vi "函数类型1测试 - 副本.vi"() -> ()   [LabVIEW 2010]
uses:
  全局量/试验配置信息.vi
panel:
  out "bRece":bool
  out "bSend":bool
  out "D_IN_1":string[][](table) caption="表格"
  in  "加载文件名称":string
  out "配置文件路径":path
  out "配置文件目录":path
  in  "同步_1":i32
  in  "数组_反馈值":dbl[][](array[numeric])
  in  "第几个数据":i32
  in  "第几组数据":i32
  in  "数组_设定值":dbl[][](array[numeric])
  in  "数组_选择":bool[](array[boolean])
  out "light_32":bool
  out "light_31":bool
  out "light_30":bool
  out "light_29":bool
  out "light_28":bool
  out "light_27":bool
  out "light_26":bool
  out "light_25":bool
  out "light_24":bool
  out "light_23":bool
  out "light_22":bool
  out "light_21":bool
  out "light_20":bool
  out "light_19":bool
  out "light_18":bool
  out "light_17":bool
  out "Analog_back":string[][](table) caption="表格"
  in  "A_32":bool
  in  "A_31":bool
  in  "A_30":bool
  in  "A_29":bool
  in  "A_28":bool
  in  "A_27":bool
  in  "A_26":bool
  in  "A_25":bool
  in  "A_24":bool
  in  "A_23":bool
  in  "A_22":bool
  in  "A_21":bool
  in  "A_20":bool
  in  "A_19":bool
  in  "A_18":bool
  in  "A_17":bool
  out "合格？":bool[][](array[boolean])
  out "测试结论":string
  out "light_16":bool
  out "light_15":bool
  out "light_14":bool
  out "light_13":bool
  out "light_12":bool
  out "light_11":bool
  out "light_10":bool
  out "light_9":bool
  out "light_8":bool
  out "light_7":bool
  out "light_6":bool
  out "light_5":bool
  out "light_4":bool
  out "light_3":bool
  out "light_2":bool
  out "light_1":bool
  out "退出？":bool
  in  "btn_反选":bool
  in  "btn_全选":bool
  in  "A_16":bool
  in  "A_15":bool
  in  "A_14":bool
  in  "A_13":bool
  in  "A_12":bool
  in  "A_11":bool
  in  "A_10":bool
  in  "A_9":bool
  in  "A_8":bool
  in  "A_7":bool
  in  "A_6":bool
  in  "A_5":bool
  in  "A_4":bool
  in  "A_3":bool
  in  "A_2":bool
  in  "A_1":bool
  in  "btn_取消":bool
  in  "btn_开始测试":bool
  in  "Analog_IN":string[][](table) caption="表格"
  out "Analog_WC":string[][](table) caption="表格"
  # "模拟量选择及输入值（V）"
  # "模拟量反馈值（V）"
  # "模拟量误差值（%）"
  # "测试结论："
  # "从0开始"
  # "从1开始,第0列没有使用"
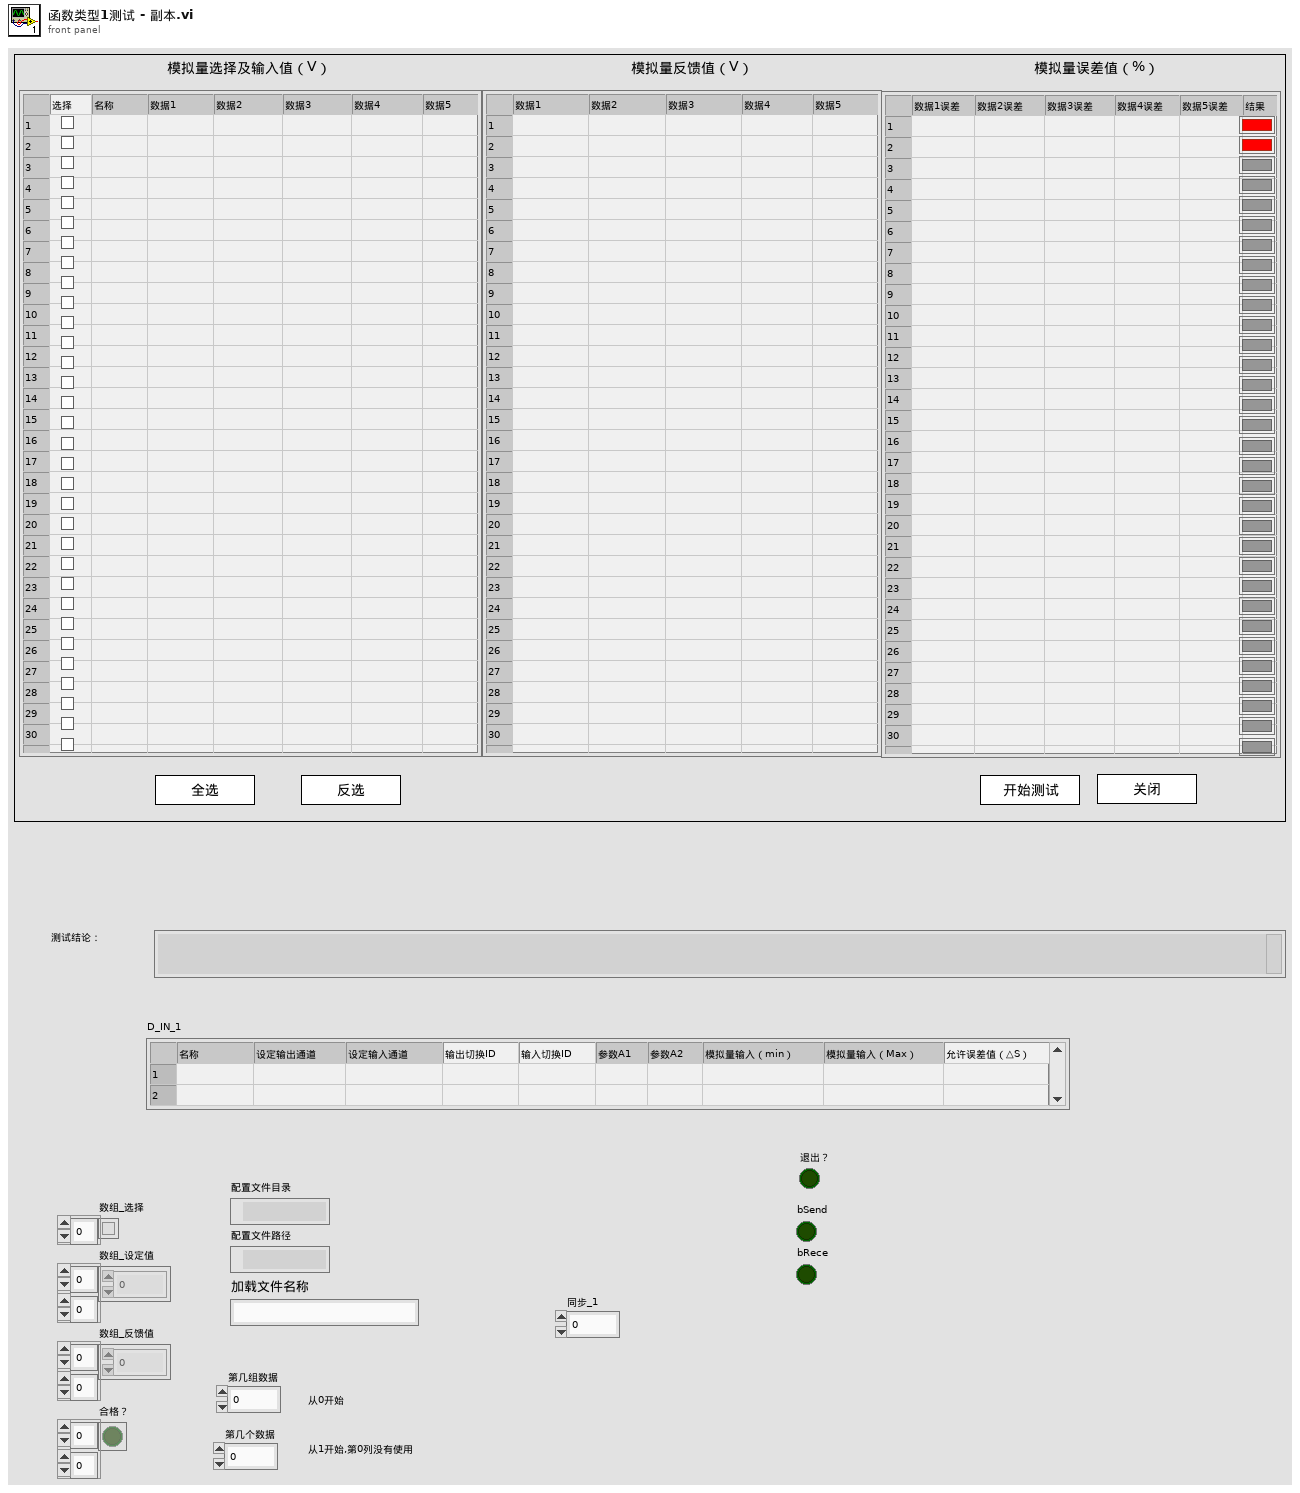
[diagram p1: front panel]
types:
  T1 = enum8{"Enabled", "Disabled", "Disabled and Grayed Out"}
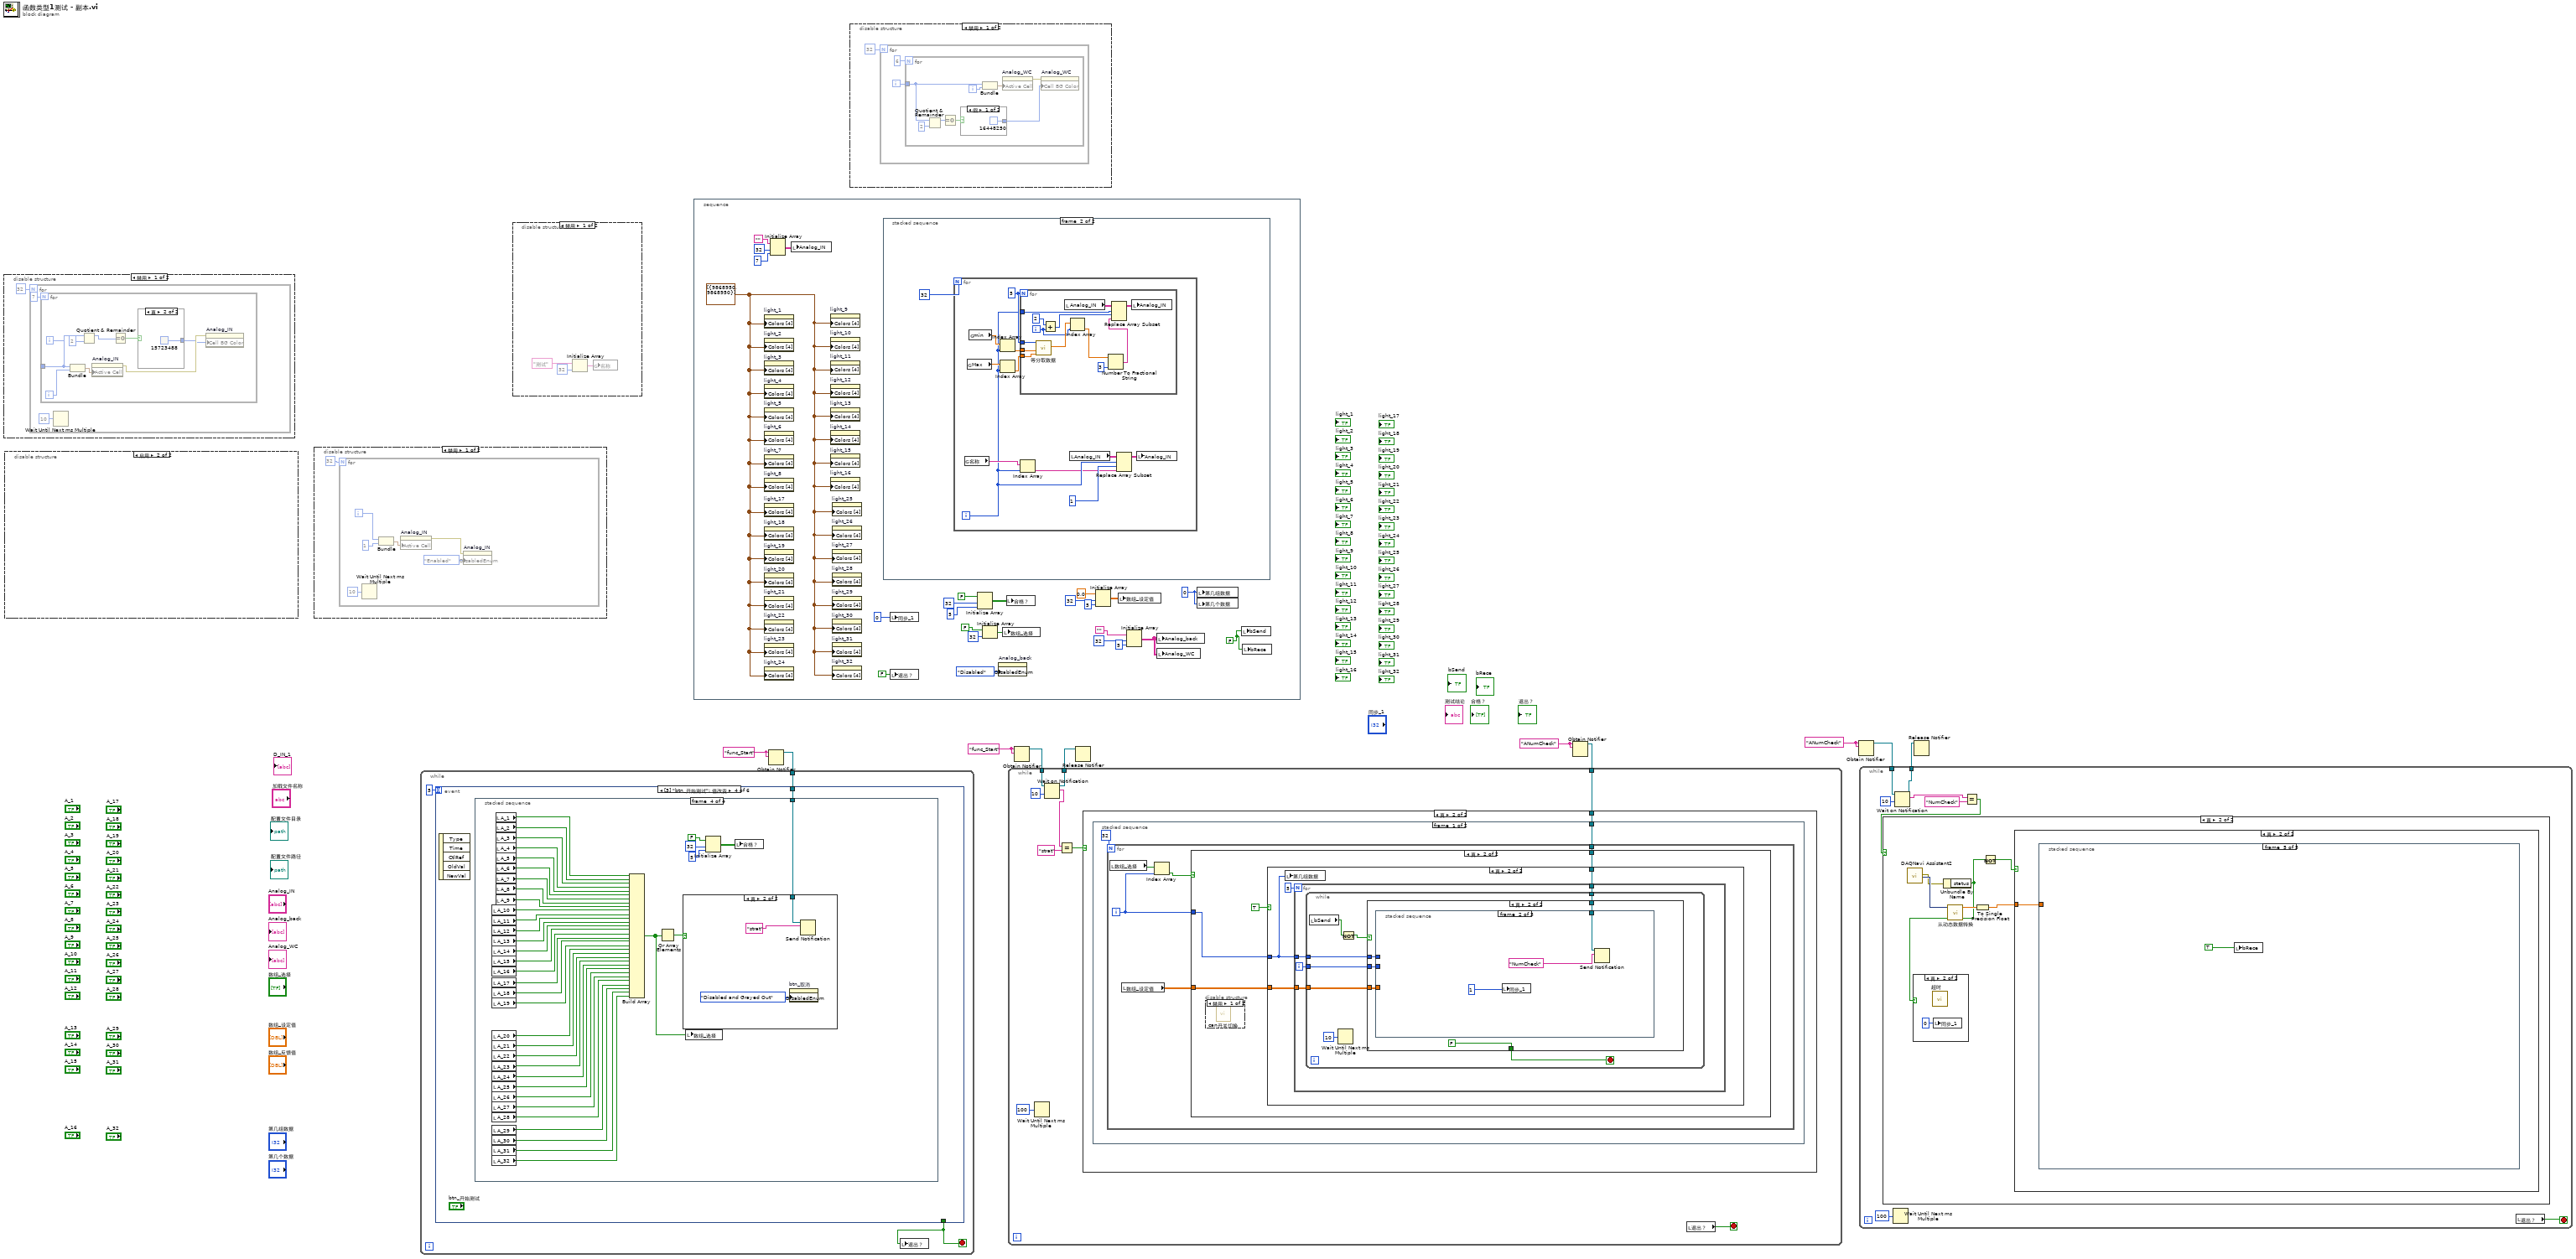
[diagram p0: block diagram]
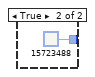
[diagram p2: hidden frame]
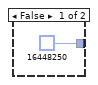
[diagram p5: hidden frame]
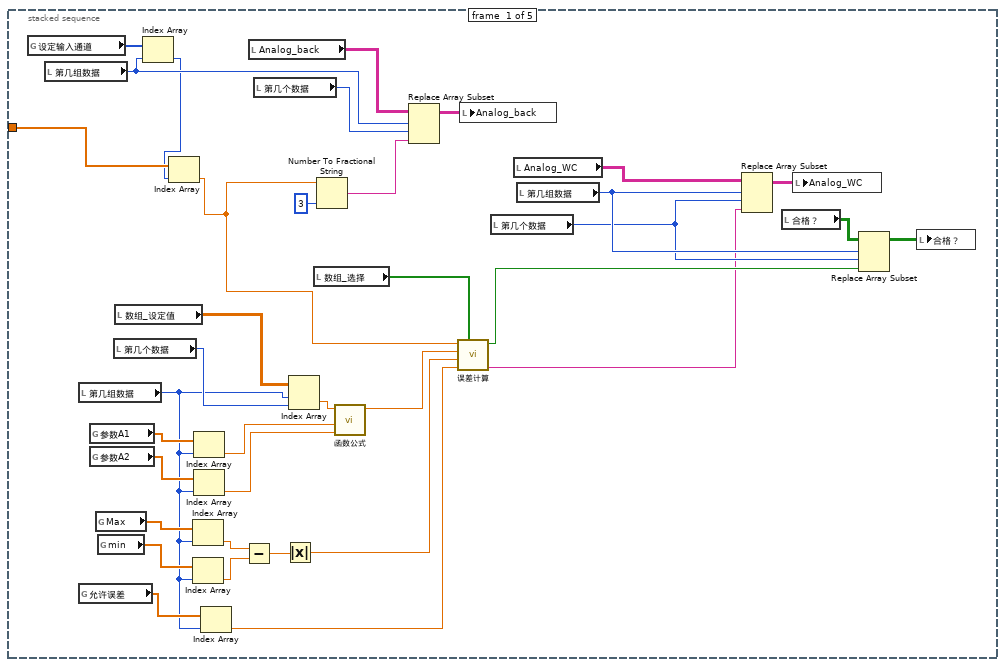
[diagram p10: hidden frame]
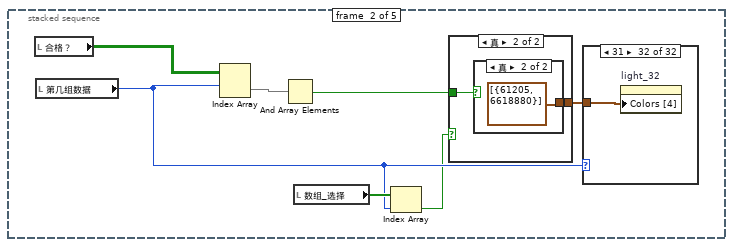
[diagram p11: hidden frame]
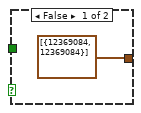
[diagram p12: hidden frame]
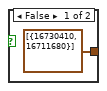
[diagram p13: hidden frame]
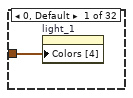
[diagram p14: hidden frame]
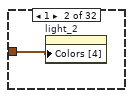
[diagram p15: hidden frame]
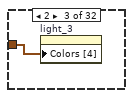
[diagram p16: hidden frame]
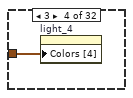
[diagram p17: hidden frame]
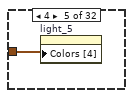
[diagram p18: hidden frame]
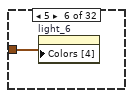
[diagram p19: hidden frame]
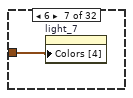
[diagram p20: hidden frame]
diagram:
  w2 = "ANumCheck" ("名称（未命名）")
  w4 = "func_Start" ("名称（未命名）")
  w8 = "ANumCheck" ("名称（未命名）")
  w10 = "func_Start" ("名称（未命名）")
  n1 = disable-structure shown="禁用" {
    frame Disabled {
      n2 = for {
        N: 32 -> [_]
        i -> [w13]
        n3 = for {
          N: 7 -> [_]
          tunnel: w13 -> [w21]
          i -> [w15]
          n4 = Bundle(w21, w15) -> (w18:cluster{i32, i32})  [unwired: 1 in]
          n5 = Quotient & Remainder(x=w21, y=2) -> (x-y*floor(x/y)=w19:i32)  [unwired: 1 out]
          n6 = property on="Analog_IN" class="Tbl (严格)"("Active Cell"=w18) -> (error out=w17:errorcluster)  [unwired: 2 in, 1 out]
          n7 = Equal To 0?(x=w19) -> (x = 0?=w22:bool)
          n8 = case shown="真" w22 {
            tunnel: [u32 16448250 u32 15723488] -> w16
            frame False {
            }
            frame True {
            }
          }
          n9 = property on="Analog_IN" class="Tbl (严格)"(error in=w17, "Cell BG Color"=w16) -> ()  [unwired: 1 in, 2 out]
        }
        n10 = Wait Until Next ms Multiple(millisecond multiple=u32 10 ("毫秒倍数")) -> ()  [unwired: 1 out]
      }
    }
    frame Enabled {
    }
  }
  n11 = disable-structure shown="启用" {
    frame Disabled {
      n12 = for {
        N: 32 -> [_]
        i -> [w26]
        n13 = for {
          N: 7 -> [_]
          tunnel: w26 -> [w29]
          i -> [w30]
          n14 = Bundle(w29, w30) -> (w33:cluster{i32, i32})  [unwired: 1 in]
          n15 = property on="Analog_IN" class="Tbl (严格)"("Active Cell"=w33) -> (error out=w31:errorcluster)  [unwired: 2 in, 1 out]
          n16 = property on="Analog_IN" class="Tbl (严格)"(error in=w31, "Justify"=enum16{"Left", "Center", "Right"}."Left" ("活动单元格:单元格对齐")) -> ()  [unwired: 1 in, 2 out]
        }
        n17 = Wait Until Next ms Multiple(millisecond multiple=u32 10 ("毫秒倍数")) -> ()  [unwired: 1 out]
      }
    }
    frame Enabled {
    }
  }
  n18 = disable-structure shown="禁用" {
    frame Disabled {
      n19 = for {
        N: 32 -> [_]
        i -> [w39]
        n20 = Wait Until Next ms Multiple(millisecond multiple=u32 10 ("毫秒倍数")) -> ()  [unwired: 1 out]
        n21 = Bundle(w39, 1) -> (w38:cluster{i32, i32})  [unwired: 1 in]
        n22 = property on="Analog_IN" class="Tbl (严格)"("Active Cell"=w38) -> (error out=w35:errorcluster)  [unwired: 2 in, 1 out]
        n23 = property on="Analog_IN" class="Tbl (严格)"(error in=w35, "DisabledEnum"=T1."Enabled" ("禁用")) -> ()  [unwired: 1 in, 2 out]
      }
    }
    frame Enabled {
    }
  }
  n24 = disable-structure shown="禁用" {
    frame Disabled {
      n25 = Initialize Array("测试", 32 ("维数大小")) -> (w42:string[])
      n26 = global write "试验配置信息.vi" "名称"(w42) -> ()
    }
    frame Enabled {
    }
  }
  n27 = stacked-sequence {
    frame #0 {
      w44 = FALSE
      w49 = 0 ("第几组数据")
      w64 = cluster{u32, u32}[] [{9868950, 9868950}]
      n28 = property on="light_1" class="Bool (严格)"("Colors [4]"=w64) -> ()  [unwired: 2 in, 2 out]
      n29 = property on="light_2" class="Bool (严格)"("Colors [4]"=w64) -> ()  [unwired: 2 in, 2 out]
      n30 = property on="light_3" class="Bool (严格)"("Colors [4]"=w64) -> ()  [unwired: 2 in, 2 out]
      n31 = property on="light_4" class="Bool (严格)"("Colors [4]"=w64) -> ()  [unwired: 2 in, 2 out]
      n32 = property on="light_5" class="Bool (严格)"("Colors [4]"=w64) -> ()  [unwired: 2 in, 2 out]
      n33 = property on="light_6" class="Bool (严格)"("Colors [4]"=w64) -> ()  [unwired: 2 in, 2 out]
      n34 = property on="light_7" class="Bool (严格)"("Colors [4]"=w64) -> ()  [unwired: 2 in, 2 out]
      n35 = property on="light_8" class="Bool (严格)"("Colors [4]"=w64) -> ()  [unwired: 2 in, 2 out]
      n36 = property on="light_17" class="Bool (严格)"("Colors [4]"=w64) -> ()  [unwired: 2 in, 2 out]
      n37 = property on="light_18" class="Bool (严格)"("Colors [4]"=w64) -> ()  [unwired: 2 in, 2 out]
      n38 = property on="light_19" class="Bool (严格)"("Colors [4]"=w64) -> ()  [unwired: 2 in, 2 out]
      n39 = property on="light_20" class="Bool (严格)"("Colors [4]"=w64) -> ()  [unwired: 2 in, 2 out]
      n40 = property on="light_21" class="Bool (严格)"("Colors [4]"=w64) -> ()  [unwired: 2 in, 2 out]
      n41 = property on="light_22" class="Bool (严格)"("Colors [4]"=w64) -> ()  [unwired: 2 in, 2 out]
      n42 = property on="light_23" class="Bool (严格)"("Colors [4]"=w64) -> ()  [unwired: 2 in, 2 out]
      n43 = property on="light_24" class="Bool (严格)"("Colors [4]"=w64) -> ()  [unwired: 2 in, 2 out]
      n44 = Initialize Array("", 32 ("维数大小"), 7 ("维数大小")) -> (w48:string[][])
      n45 = local write "Analog_IN"(w48) -> ()
      n46 = property on="light_9" class="Bool (严格)"("Colors [4]"=w64) -> ()  [unwired: 2 in, 2 out]
      n47 = property on="light_10" class="Bool (严格)"("Colors [4]"=w64) -> ()  [unwired: 2 in, 2 out]
      n48 = property on="light_11" class="Bool (严格)"("Colors [4]"=w64) -> ()  [unwired: 2 in, 2 out]
      n49 = property on="light_12" class="Bool (严格)"("Colors [4]"=w64) -> ()  [unwired: 2 in, 2 out]
      n50 = property on="light_13" class="Bool (严格)"("Colors [4]"=w64) -> ()  [unwired: 2 in, 2 out]
      n51 = property on="light_14" class="Bool (严格)"("Colors [4]"=w64) -> ()  [unwired: 2 in, 2 out]
      n52 = property on="light_15" class="Bool (严格)"("Colors [4]"=w64) -> ()  [unwired: 2 in, 2 out]
      n53 = property on="light_16" class="Bool (严格)"("Colors [4]"=w64) -> ()  [unwired: 2 in, 2 out]
      n54 = property on="light_25" class="Bool (严格)"("Colors [4]"=w64) -> ()  [unwired: 2 in, 2 out]
      n55 = property on="light_26" class="Bool (严格)"("Colors [4]"=w64) -> ()  [unwired: 2 in, 2 out]
      n56 = property on="light_27" class="Bool (严格)"("Colors [4]"=w64) -> ()  [unwired: 2 in, 2 out]
      n57 = property on="light_28" class="Bool (严格)"("Colors [4]"=w64) -> ()  [unwired: 2 in, 2 out]
      n58 = property on="light_29" class="Bool (严格)"("Colors [4]"=w64) -> ()  [unwired: 2 in, 2 out]
      n59 = property on="light_30" class="Bool (严格)"("Colors [4]"=w64) -> ()  [unwired: 2 in, 2 out]
      n60 = property on="light_31" class="Bool (严格)"("Colors [4]"=w64) -> ()  [unwired: 2 in, 2 out]
      n61 = property on="light_32" class="Bool (严格)"("Colors [4]"=w64) -> ()  [unwired: 2 in, 2 out]
      n62 = stacked-sequence {
        frame #0 {
          n63 = for {
            N: 32 ("维数大小") -> [_]
            tunnel: [w109] -> w73 mode=indexing
            tunnel: [w105] -> w72 mode=indexing
            tunnel: [w103] -> w71 mode=indexing
            tunnel: [w100] -> w70 mode=indexing
            tunnel: [w97] -> w69 mode=indexing
            tunnel: [w94] -> w75 mode=indexing
            tunnel: [w91] -> w76 mode=indexing
            tunnel: [w88] -> w77 mode=indexing
            tunnel: [w85] -> w78 mode=indexing
            tunnel: [w81] -> w79 mode=indexing
            i -> [w83]
            n64 = global read "试验配置信息.vi" "D_IN_1"() -> (w80:string[][])
            n65 = Index Array(array=w80, index (row)=w83, index (col)=0 ("禁用的索引 (列)")) -> (element=w109:string)
            n66 = Index Array(array=w80, index (row)=w83, index (col)=2 ("禁用的索引 (列)")) -> (element=w99:string)
            n67 = Index Array(array=w80, index (row)=w83, index (col)=3 ("禁用的索引 (列)")) -> (element=w95:string)
            n68 = Index Array(array=w80, index (row)=w83, index (col)=4 ("禁用的索引 (列)")) -> (element=w93:string)
            n69 = Index Array(array=w80, index (row)=w83, index (col)=5 ("禁用的索引 (列)")) -> (element=w90:string)
            n70 = Index Array(array=w80, index (row)=w83, index (col)=9 ("禁用的索引 (列)")) -> (element=w82:string)
            n71 = Index Array(array=w80, index (row)=w83, index (col)=1 ("禁用的索引 (列)")) -> (element=w102:string)
            n72 = Index Array(array=w80, index (row)=w83, index (col)=6 ("禁用的索引 (列)")) -> (element=w86:string)
            n73 = Index Array(array=w80, index (row)=w83, index (col)=7 ("禁用的索引 (列)")) -> (element=w106:string)
            n74 = Index Array(array=w80, index (row)=w83, index (col)=8 ("禁用的索引 (列)")) -> (element=w104:string)
            n75 = Decimal String To Number(string=w99) -> (number=w97:i32)  [unwired: 2 in, 1 out]
            n76 = Decimal String To Number(string=w95) -> (number=w94:i32)  [unwired: 2 in, 1 out]
            n77 = Decimal String To Number(string=w93) -> (number=w91:i32)  [unwired: 2 in, 1 out]
            n78 = Decimal String To Number(string=w102) -> (number=w100:i32)  [unwired: 2 in, 1 out]
            n79 = Fract/Exp String To Number(string=w90) -> (number=w88:dbl)  [unwired: 3 in, 1 out]
            n80 = Fract/Exp String To Number(string=w82) -> (number=w81:dbl)  [unwired: 3 in, 1 out]
            n81 = Fract/Exp String To Number(string=w86) -> (number=w85:dbl)  [unwired: 3 in, 1 out]
            n82 = Fract/Exp String To Number(string=w106) -> (number=w105:dbl)  [unwired: 3 in, 1 out]
            n83 = Fract/Exp String To Number(string=w104) -> (number=w103:dbl)  [unwired: 3 in, 1 out]
          }
          n84 = global write "试验配置信息.vi" "名称"(w73) -> ()
          n85 = global write "试验配置信息.vi" "设定输入通道"(w69) -> ()
          n86 = global write "试验配置信息.vi" "输出切换ID"(w75) -> ()
          n87 = global write "试验配置信息.vi" "输入切换ID"(w76) -> ()
          n88 = global write "试验配置信息.vi" "参数A1"(w77) -> ()
          n89 = global write "试验配置信息.vi" "允许误差"(w79) -> ()
          n90 = global write "试验配置信息.vi" "设定输出通道"(w70) -> ()
          n91 = global write "试验配置信息.vi" "参数A2"(w78) -> ()
          n92 = global write "试验配置信息.vi" "min"(w72) -> ()
          n93 = global write "试验配置信息.vi" "Max"(w71) -> ()
        }
        frame #1 {
          n94 = for {
            N: 32 -> [_]
            i -> [w114]
            w118 = 5 ("num")
            n95 = global read "试验配置信息.vi" "名称"() -> (w117:string[])
            n96 = global read "试验配置信息.vi" "Max"() -> (w121:dbl[])
            n97 = global read "试验配置信息.vi" "min"() -> (w122:dbl[])
            n98 = Index Array(array=w122, index=w114) -> (element=w120:dbl)
            n99 = Index Array(array=w121, index=w114) -> (element=w119:dbl)
            n100 = for {
              N: w118 -> [_]
              tunnel: w114 -> [w133]
              tunnel: w120 -> [w130]
              tunnel: w119 -> [w129]
              tunnel: w118 -> [w128]
              i -> [w126]
              n101 = call "等分取数据.vi"("Max"=w129, "MIN"=w130, "num"=w128) -> ("数据点"=w127:dbl[])  [unwired: 5 in]
              n102 = Add(x=2, y=w126) -> (x+y=w131:i32)
              n103 = local read "Analog_IN"() -> (w135:string[][])
              n104 = Index Array(array=w127, index=w126) -> (element=w124:dbl)
              n105 = Number To Fractional String(number=w124, precision (6)=i16 3 ("精度(6)")) -> (F-format string=w125:string)  [unwired: 2 in]
              n106 = Replace Array Subset(array=w135, new element=w125, index (row)=w133, index (col)=w131) -> (w134:string[][])
              n107 = local write "Analog_IN"(w134) -> ()
            }
            n108 = Index Array(array=w117, index=w114) -> (element=w112:string)
            n109 = local read "Analog_IN"() -> (w115:string[][])
            n110 = Replace Array Subset(array=w115, new element=w112, index (row)=w114, index (col)=1) -> (w116:string[][])
            n111 = local write "Analog_IN"(w116) -> ()
          }
        }
      }
      n112 = local write "同步_1"(0 ("同步_2")) -> ()
      n113 = local write "退出？"(FALSE ("退出？")) -> ()
      n114 = Initialize Array(FALSE, 32 ("维数大小"), 5 ("维数大小")) -> (w65:bool[][])
      n115 = Initialize Array(FALSE, 32 ("维数大小")) -> (w53:bool[])
      n116 = property on="Analog_back" class="Tbl (严格)"("DisabledEnum"=T1."Disabled" ("禁用")) -> ()  [unwired: 2 in, 2 out]
      n117 = local write "数组_选择"(w53) -> ()
      n118 = local write "合格？"(w65) -> ()
      n119 = Initialize Array(0.0, 32 ("维数大小"), 5 ("维数大小")) -> (w56:dbl[][])
      n120 = local write "数组_设定值"(w56) -> ()
      n121 = Initialize Array("", 32 ("维数大小"), 5 ("维数大小")) -> (w60:string[][])
      n122 = local write "Analog_back"(w60) -> ()
      n123 = local write "Analog_WC"(w60) -> ()
      n124 = local write "第几组数据"(w49) -> ()
      n125 = local write "第几个数据"(w49) -> ()
      n126 = local write "bSend"(w44) -> ()
      n127 = local write "bRece"(w44) -> ()
    }
  }
  n128 = Obtain Notifier(name (unnamed)=w10, notification data type=w10) -> (notifier out=w7:refnum<notifier>)  [unwired: 2 in, 2 out]
  n129 = while {
    tunnel: w7 -> [w137]
    stop <- w138 stop-if-true
    n130 = event shown="[3] \"btn_开始测试\": 值改变" {
      selector: _ -> [_ _ _ _ _ _]
      dyn-events: _ -> [_ _ _ _ _ _]
      timeout: 5 -> [_ _ _ _ _ _]
      tunnel: [_ TRUE TRUE _ _ _] -> w138
      tunnel: w137 -> [_ _ _ w142 _ _]
      event Timeout {
        n131 = event-data() -> ()  [unwired: 1 in, 2 out]
        n132 = Wait Until Next ms Multiple(millisecond multiple=u32 2 ("毫秒倍数")) -> ()  [unwired: 1 out]
      }
      event Panel Close {
        n133 = event-data() -> ()  [unwired: 1 in, 3 out]
      }
      event "btn_取消": Value Change {
        n134 = event-data() -> ()  [unwired: 1 in, 5 out]
      }
      event "btn_开始测试": Value Change {
        n135 = event-data() -> ()  [unwired: 1 in, 5 out]
        n136 = stacked-sequence {
          tunnel: w142 -> [_ _ _ w225]
          frame #0 {
            w143 = FALSE
            w148 = 0 ("第几组数据")
            # "测试期间不准退出防止程序卡死"
            n137 = local read "Analog_IN"() -> (w154:string[][])
            n138 = Delete From Array(array=w154, length=1 ("长度"), index (col)=0 ("禁用的索引 (列)")) -> (array with subset deleted=w146:string[][])  [unwired: 1 in, 1 out]
            n139 = Delete From Array(array=w146, length=1 ("长度"), index (col)=0 ("禁用的索引 (列)")) -> (array with subset deleted=w144:string[][])  [unwired: 1 in, 1 out]
            n140 = for {
              N: 32 -> [_]
              tunnel: w144 -> [w157] mode=indexing
              tunnel: [w156] -> w153 mode=indexing
              n141 = for {
                N: 5 -> [_]
                tunnel: w157 -> [w159] mode=indexing
                tunnel: [w158] -> w156 mode=indexing
                n142 = Fract/Exp String To Number(string=w159) -> (number=w158:dbl)  [unwired: 3 in, 1 out]
              }
            }
            n143 = local write "第几组数据"(w148) -> ()
            n144 = local write "第几个数据"(w148) -> ()
            n145 = local write "同步_1"(0 ("同步_2")) -> ()
            n146 = local write "数组_设定值"(w153) -> ()
            n147 = local write "bSend"(w143) -> ()
            n148 = local write "bRece"(w143) -> ()
          }
          frame #1 {
            n149 = local read "Analog_back"() -> (w162:string[][])
            n150 = local read "Analog_WC"() -> (w161:string[][])
            n151 = for {
              tunnel: w161 -> [w198] mode=indexing
              i -> [w197]
              n152 = for {
                tunnel: w198 -> [_] mode=indexing
                tunnel: w197 -> [w202]
                i -> [w201]
                n153 = local read "Analog_WC"() -> (w203:string[][])
                n154 = Replace Array Subset(array=w203, new element="", index (row)=w202, index (col)=w201) -> (w199:string[][])
                n155 = local write "Analog_WC"(w199) -> ()
              }
            }
            n156 = for {
              tunnel: w162 -> [w205] mode=indexing
              i -> [w204]
              n157 = for {
                tunnel: w205 -> [_] mode=indexing
                tunnel: w204 -> [w209]
                i -> [w208]
                n158 = local read "Analog_back"() -> (w210:string[][])
                n159 = Replace Array Subset(array=w210, new element="", index (row)=w209, index (col)=w208) -> (w206:string[][])
                n160 = local write "Analog_back"(w206) -> ()
              }
            }
            n161 = for {
              N: 32 -> [_]
              i -> [w164]
              n162 = case shown="31" w164 {
                tunnel: cluster{u32, u32}[] [{9868950, 9868950}] -> [w165 w166 w167 w168 w169 w170 w171 w172 w173 w174 w175 w176 w177 w178 w179 w180 w181 w182 w183 w184 w185 w186 w187 w188 w189 w190 w191 w192 w193 w194 w195 w196]
                frame 0, Default {
                  n163 = property on="light_1" class="Bool (严格)"("Colors [4]"=w165) -> ()  [unwired: 2 in, 2 out]
                }
                frame 1 {
                  n164 = property on="light_2" class="Bool (严格)"("Colors [4]"=w166) -> ()  [unwired: 2 in, 2 out]
                }
                frame 2 {
                  n165 = property on="light_3" class="Bool (严格)"("Colors [4]"=w167) -> ()  [unwired: 2 in, 2 out]
                }
                frame 3 {
                  n166 = property on="light_4" class="Bool (严格)"("Colors [4]"=w168) -> ()  [unwired: 2 in, 2 out]
                }
                frame 4 {
                  n167 = property on="light_5" class="Bool (严格)"("Colors [4]"=w169) -> ()  [unwired: 2 in, 2 out]
                }
                frame 5 {
                  n168 = property on="light_6" class="Bool (严格)"("Colors [4]"=w170) -> ()  [unwired: 2 in, 2 out]
                }
                frame 6 {
                  n169 = property on="light_7" class="Bool (严格)"("Colors [4]"=w171) -> ()  [unwired: 2 in, 2 out]
                }
                frame 7 {
                  n170 = property on="light_8" class="Bool (严格)"("Colors [4]"=w172) -> ()  [unwired: 2 in, 2 out]
                }
                frame 8 {
                  n171 = property on="light_9" class="Bool (严格)"("Colors [4]"=w173) -> ()  [unwired: 2 in, 2 out]
                }
                frame 9 {
                  n172 = property on="light_10" class="Bool (严格)"("Colors [4]"=w174) -> ()  [unwired: 2 in, 2 out]
                }
                frame 10 {
                  n173 = property on="light_11" class="Bool (严格)"("Colors [4]"=w175) -> ()  [unwired: 2 in, 2 out]
                }
                frame 11 {
                  n174 = property on="light_12" class="Bool (严格)"("Colors [4]"=w176) -> ()  [unwired: 2 in, 2 out]
                }
                frame 12 {
                  n175 = property on="light_13" class="Bool (严格)"("Colors [4]"=w177) -> ()  [unwired: 2 in, 2 out]
                }
                frame 13 {
                  n176 = property on="light_14" class="Bool (严格)"("Colors [4]"=w178) -> ()  [unwired: 2 in, 2 out]
                }
                frame 14 {
                  n177 = property on="light_15" class="Bool (严格)"("Colors [4]"=w179) -> ()  [unwired: 2 in, 2 out]
                }
                frame 15 {
                  n178 = property on="light_16" class="Bool (严格)"("Colors [4]"=w180) -> ()  [unwired: 2 in, 2 out]
                }
                frame 16 {
                  n179 = property on="light_17" class="Bool (严格)"("Colors [4]"=w181) -> ()  [unwired: 2 in, 2 out]
                }
                frame 17 {
                  n180 = property on="light_18" class="Bool (严格)"("Colors [4]"=w182) -> ()  [unwired: 2 in, 2 out]
                }
                frame 18 {
                  n181 = property on="light_19" class="Bool (严格)"("Colors [4]"=w183) -> ()  [unwired: 2 in, 2 out]
                }
                frame 19 {
                  n182 = property on="light_20" class="Bool (严格)"("Colors [4]"=w184) -> ()  [unwired: 2 in, 2 out]
                }
                frame 20 {
                  n183 = property on="light_21" class="Bool (严格)"("Colors [4]"=w185) -> ()  [unwired: 2 in, 2 out]
                }
                frame 21 {
                  n184 = property on="light_22" class="Bool (严格)"("Colors [4]"=w186) -> ()  [unwired: 2 in, 2 out]
                }
                frame 22 {
                  n185 = property on="light_23" class="Bool (严格)"("Colors [4]"=w187) -> ()  [unwired: 2 in, 2 out]
                }
                frame 23 {
                  n186 = property on="light_24" class="Bool (严格)"("Colors [4]"=w188) -> ()  [unwired: 2 in, 2 out]
                }
                frame 24 {
                  n187 = property on="light_25" class="Bool (严格)"("Colors [4]"=w189) -> ()  [unwired: 2 in, 2 out]
                }
                frame 25 {
                  n188 = property on="light_26" class="Bool (严格)"("Colors [4]"=w190) -> ()  [unwired: 2 in, 2 out]
                }
                frame 26 {
                  n189 = property on="light_27" class="Bool (严格)"("Colors [4]"=w191) -> ()  [unwired: 2 in, 2 out]
                }
                frame 27 {
                  n190 = property on="light_28" class="Bool (严格)"("Colors [4]"=w192) -> ()  [unwired: 2 in, 2 out]
                }
                frame 28 {
                  n191 = property on="light_29" class="Bool (严格)"("Colors [4]"=w193) -> ()  [unwired: 2 in, 2 out]
                }
                frame 29 {
                  n192 = property on="light_30" class="Bool (严格)"("Colors [4]"=w194) -> ()  [unwired: 2 in, 2 out]
                }
                frame 30 {
                  n193 = property on="light_31" class="Bool (严格)"("Colors [4]"=w195) -> ()  [unwired: 2 in, 2 out]
                }
                frame 31 {
                  n194 = property on="light_32" class="Bool (严格)"("Colors [4]"=w196) -> ()  [unwired: 2 in, 2 out]
                }
              }
            }
          }
          frame #2 {
            n195 = for {
              N: 32 -> [_]
              i -> [w213]
              n196 = disable-structure shown="禁用" {
                frame Disabled {
                  n197 = Wait Until Next ms Multiple(millisecond multiple=u32 10 ("毫秒倍数")) -> ()  [unwired: 1 out]
                }
                frame Enabled {
                }
              }
              n198 = for {
                N: 6 -> [_]
                tunnel: w213 -> [w221]
                i -> [w218]
                n199 = Quotient & Remainder(x=w221, y=2) -> (x-y*floor(x/y)=w219:i32)  [unwired: 1 out]
                n200 = Equal To 0?(x=w219) -> (x = 0?=w222:bool)
                n201 = case shown="假" w222 {
                  tunnel: [u32 16448250 u32 15723488] -> w215
                  frame False {
                  }
                  frame True {
                  }
                }
                n202 = Bundle(w221, w218) -> (w217:cluster{i32, i32})  [unwired: 1 in]
                n203 = property on="Analog_WC" class="Tbl (严格)"("Active Cell"=w217) -> (error out=w216:errorcluster)  [unwired: 2 in, 1 out]
                n204 = property on="Analog_WC" class="Tbl (严格)"(error in=w216, "Cell BG Color"=w215) -> ()  [unwired: 1 in, 2 out]
              }
            }
          }
          frame #3 {
            n205 = local read "A_10"() -> (w254:bool)
            n206 = local read "A_11"() -> (w253:bool)
            n207 = local read "A_12"() -> (w252:bool)
            n208 = local read "A_13"() -> (w251:bool)
            n209 = local read "A_14"() -> (w250:bool)
            n210 = local read "A_15"() -> (w249:bool)
            n211 = local read "A_16"() -> (w248:bool)
            n212 = local read "A_17"() -> (w247:bool)
            n213 = local read "A_18"() -> (w246:bool)
            n214 = local read "A_19"() -> (w245:bool)
            n215 = local read "A_20"() -> (w244:bool)
            n216 = local read "A_21"() -> (w243:bool)
            n217 = local read "A_22"() -> (w242:bool)
            n218 = local read "A_23"() -> (w241:bool)
            n219 = local read "A_24"() -> (w240:bool)
            n220 = local read "A_25"() -> (w239:bool)
            n221 = local read "A_26"() -> (w238:bool)
            n222 = local read "A_27"() -> (w237:bool)
            n223 = local read "A_28"() -> (w236:bool)
            n224 = local read "A_29"() -> (w235:bool)
            n225 = local read "A_30"() -> (w234:bool)
            n226 = local read "A_31"() -> (w233:bool)
            n227 = local read "A_32"() -> (w232:bool)
            n228 = local read "A_1"() -> (w263:bool)
            n229 = local read "A_2"() -> (w262:bool)
            n230 = local read "A_3"() -> (w261:bool)
            n231 = local read "A_4"() -> (w260:bool)
            n232 = local read "A_5"() -> (w259:bool)
            n233 = local read "A_6"() -> (w258:bool)
            n234 = local read "A_7"() -> (w257:bool)
            n235 = local read "A_8"() -> (w256:bool)
            n236 = local read "A_9"() -> (w255:bool)
            n237 = Build Array(w263, w262, w261, w260, w259, w258, w257, w256, w255, w254, w253, w252, w251, w250, w249, w248, w247, w246, w245, w244, w243, w242, w241, w240, w239, w238, w237, w236, w235, w234, w233, w232) -> (w226:bool[])
            n238 = Or Array Elements(Boolean array=w226) -> (logical OR=w231:bool)
            n239 = case shown="真" w231 {
              tunnel: w225 -> [_ w265]
              frame False {
                n240 = call "显示对话框信息"() -> ()  [unwired: 10 in, 2 out]
              }
              frame True {
                n241 = property on="btn_取消" class="Bool"("DisabledEnum"=T1."Disabled and Grayed Out" ("禁用")) -> ()  [unwired: 2 in, 2 out]
                n242 = Send Notification(notification="strat" ("通知"), notifier=w265) -> ()  [unwired: 1 in, 2 out]
              }
            }
            n243 = local write "数组_选择"(w226) -> ()
            n244 = Initialize Array(FALSE, 32 ("维数大小"), 5 ("维数大小")) -> (w227:bool[][])
            n245 = local write "合格？"(w227) -> ()
          }
        }
      }
      event "btn_全选": Value Change {
        w267 = TRUE ("单选_AD_1")
        n246 = event-data() -> ()  [unwired: 1 in, 5 out]
        n247 = local write "A_1"(w267) -> ()
        n248 = local write "A_2"(w267) -> ()
        n249 = local write "A_3"(w267) -> ()
        n250 = local write "A_4"(w267) -> ()
        n251 = local write "A_5"(w267) -> ()
        n252 = local write "A_6"(w267) -> ()
        n253 = local write "A_7"(w267) -> ()
        n254 = local write "A_8"(w267) -> ()
        n255 = local write "A_9"(w267) -> ()
        n256 = local write "A_10"(w267) -> ()
        n257 = local write "A_11"(w267) -> ()
        n258 = local write "A_12"(w267) -> ()
        n259 = local write "A_13"(w267) -> ()
        n260 = local write "A_14"(w267) -> ()
        n261 = local write "A_15"(w267) -> ()
        n262 = local write "A_16"(w267) -> ()
        n263 = local write "A_17"(w267) -> ()
        n264 = local write "A_18"(w267) -> ()
        n265 = local write "A_19"(w267) -> ()
        n266 = local write "A_20"(w267) -> ()
        n267 = local write "A_21"(w267) -> ()
        n268 = local write "A_22"(w267) -> ()
        n269 = local write "A_23"(w267) -> ()
        n270 = local write "A_24"(w267) -> ()
        n271 = local write "A_25"(w267) -> ()
        n272 = local write "A_26"(w267) -> ()
        n273 = local write "A_27"(w267) -> ()
        n274 = local write "A_28"(w267) -> ()
        n275 = local write "A_29"(w267) -> ()
        n276 = local write "A_30"(w267) -> ()
        n277 = local write "A_31"(w267) -> ()
        n278 = local write "A_32"(w267) -> ()
      }
      event "btn_反选": Value Change {
        n279 = event-data() -> ()  [unwired: 1 in, 5 out]
        n280 = local read "A_17"() -> (w299:bool)
        n281 = local read "A_18"() -> (w297:bool)
        n282 = local read "A_19"() -> (w295:bool)
        n283 = local read "A_20"() -> (w293:bool)
        n284 = local read "A_21"() -> (w291:bool)
        n285 = local read "A_22"() -> (w289:bool)
        n286 = local read "A_23"() -> (w287:bool)
        n287 = local read "A_24"() -> (w285:bool)
        n288 = local read "A_25"() -> (w283:bool)
        n289 = local read "A_26"() -> (w281:bool)
        n290 = local read "A_27"() -> (w279:bool)
        n291 = local read "A_28"() -> (w277:bool)
        n292 = local read "A_29"() -> (w275:bool)
        n293 = local read "A_30"() -> (w273:bool)
        n294 = local read "A_31"() -> (w271:bool)
        n295 = local read "A_32"() -> (w269:bool)
        n296 = local read "A_1"() -> (w331:bool)
        n297 = local read "A_2"() -> (w329:bool)
        n298 = local read "A_3"() -> (w328:bool)
        n299 = local read "A_4"() -> (w327:bool)
        n300 = local read "A_5"() -> (w326:bool)
        n301 = local read "A_6"() -> (w325:bool)
        n302 = local read "A_7"() -> (w324:bool)
        n303 = local read "A_8"() -> (w323:bool)
        n304 = local read "A_9"() -> (w322:bool)
        n305 = local read "A_10"() -> (w321:bool)
        n306 = local read "A_11"() -> (w320:bool)
        n307 = local read "A_12"() -> (w319:bool)
        n308 = local read "A_13"() -> (w318:bool)
        n309 = local read "A_14"() -> (w317:bool)
        n310 = local read "A_15"() -> (w316:bool)
        n311 = local read "A_16"() -> (w315:bool)
        n312 = Not(x=w331) -> (.not. x?=w330:bool)
        n313 = Not(x=w329) -> (.not. x?=w300:bool)
        n314 = Not(x=w328) -> (.not. x?=w301:bool)
        n315 = Not(x=w327) -> (.not. x?=w302:bool)
        n316 = Not(x=w326) -> (.not. x?=w303:bool)
        n317 = Not(x=w325) -> (.not. x?=w304:bool)
        n318 = Not(x=w324) -> (.not. x?=w305:bool)
        n319 = Not(x=w323) -> (.not. x?=w306:bool)
        n320 = Not(x=w322) -> (.not. x?=w307:bool)
        n321 = Not(x=w321) -> (.not. x?=w308:bool)
        n322 = Not(x=w320) -> (.not. x?=w309:bool)
        n323 = Not(x=w319) -> (.not. x?=w310:bool)
        n324 = Not(x=w318) -> (.not. x?=w311:bool)
        n325 = Not(x=w317) -> (.not. x?=w312:bool)
        n326 = Not(x=w316) -> (.not. x?=w313:bool)
        n327 = Not(x=w315) -> (.not. x?=w314:bool)
        n328 = Not(x=w299) -> (.not. x?=w298:bool)
        n329 = Not(x=w297) -> (.not. x?=w296:bool)
        n330 = Not(x=w295) -> (.not. x?=w294:bool)
        n331 = Not(x=w293) -> (.not. x?=w292:bool)
        n332 = Not(x=w291) -> (.not. x?=w290:bool)
        n333 = Not(x=w289) -> (.not. x?=w288:bool)
        n334 = Not(x=w287) -> (.not. x?=w286:bool)
        n335 = Not(x=w285) -> (.not. x?=w284:bool)
        n336 = Not(x=w283) -> (.not. x?=w282:bool)
        n337 = Not(x=w281) -> (.not. x?=w280:bool)
        n338 = Not(x=w279) -> (.not. x?=w278:bool)
        n339 = Not(x=w277) -> (.not. x?=w276:bool)
        n340 = Not(x=w275) -> (.not. x?=w274:bool)
        n341 = Not(x=w273) -> (.not. x?=w272:bool)
        n342 = Not(x=w271) -> (.not. x?=w270:bool)
        n343 = Not(x=w269) -> (.not. x?=w268:bool)
        n344 = local write "A_1"(w330) -> ()
        n345 = local write "A_2"(w300) -> ()
        n346 = local write "A_3"(w301) -> ()
        n347 = local write "A_4"(w302) -> ()
        n348 = local write "A_5"(w303) -> ()
        n349 = local write "A_6"(w304) -> ()
        n350 = local write "A_7"(w305) -> ()
        n351 = local write "A_8"(w306) -> ()
        n352 = local write "A_9"(w307) -> ()
        n353 = local write "A_10"(w308) -> ()
        n354 = local write "A_11"(w309) -> ()
        n355 = local write "A_12"(w310) -> ()
        n356 = local write "A_13"(w311) -> ()
        n357 = local write "A_14"(w312) -> ()
        n358 = local write "A_15"(w313) -> ()
        n359 = local write "A_16"(w314) -> ()
        n360 = local write "A_17"(w298) -> ()
        n361 = local write "A_18"(w296) -> ()
        n362 = local write "A_19"(w294) -> ()
        n363 = local write "A_20"(w292) -> ()
        n364 = local write "A_21"(w290) -> ()
        n365 = local write "A_22"(w288) -> ()
        n366 = local write "A_23"(w286) -> ()
        n367 = local write "A_24"(w284) -> ()
        n368 = local write "A_25"(w282) -> ()
        n369 = local write "A_26"(w280) -> ()
        n370 = local write "A_27"(w278) -> ()
        n371 = local write "A_28"(w276) -> ()
        n372 = local write "A_29"(w274) -> ()
        n373 = local write "A_30"(w272) -> ()
        n374 = local write "A_31"(w270) -> ()
        n375 = local write "A_32"(w268) -> ()
      }
    }
    n376 = local write "退出？"(w138) -> ()
  }
  n377 = disable-structure shown="禁用" {
    frame Disabled {
      n378 = for {
        N: 32 -> [_]
        i -> [w334]
        n379 = for {
          N: 6 -> [_]
          tunnel: w334 -> [w341]
          i -> [w338]
          n380 = Quotient & Remainder(x=w341, y=2) -> (x-y*floor(x/y)=w339:i32)  [unwired: 1 out]
          n381 = Equal To 0?(x=w339) -> (x = 0?=w342:bool)
          n382 = case shown="假" w342 {
            tunnel: [u32 16448250 u32 15723488] -> w335
            frame False {
            }
            frame True {
            }
          }
          n383 = Bundle(w341, w338) -> (w337:cluster{i32, i32})  [unwired: 1 in]
          n384 = property on="Analog_WC" class="Tbl (严格)"("Active Cell"=w337) -> (error out=w336:errorcluster)  [unwired: 2 in, 1 out]
          n385 = property on="Analog_WC" class="Tbl (严格)"(error in=w336, "Cell BG Color"=w335) -> ()  [unwired: 1 in, 2 out]
        }
      }
    }
    frame Enabled {
    }
  }
  n386 = Obtain Notifier(name (unnamed)=w4, notification data type=w4) -> (notifier out=w3:refnum<notifier>)  [unwired: 2 in, 2 out]
  n387 = Obtain Notifier(name (unnamed)=w8, notification data type=w8) -> (notifier out=w6:refnum<notifier>)  [unwired: 2 in, 2 out]
  n388 = while {
    tunnel: [w349] -> w9
    tunnel: w6 -> [w347]
    tunnel: w3 -> [w346]
    stop <- w352 stop-if-true
    n389 = Wait Until Next ms Multiple(millisecond multiple=u32 100 ("毫秒倍数")) -> ()  [unwired: 1 out]
    n390 = Wait on Notification(notifier=w346, timeout in ms (-1)=10 ("超时毫秒(-1)")) -> (notifier out=w349:refnum<notifier>, notification=w348:string)  [unwired: 2 in, 2 out]
    n391 = Equal?(x=w348, y="strat" ("通知")) -> (x = y?=w350:bool)
    n392 = case shown="真" w350 {
      tunnel: w347 -> [_ w354]
      frame False {
      }
      frame True {
        n393 = stacked-sequence {
          tunnel: w354 -> [w355 _]
          frame #0 {
            n394 = for {
              N: 32 -> [_]
              tunnel: w355 -> [w357]
              i -> [w359]
              n395 = local read "数组_选择"() -> (w360:bool[])
              n396 = local read "数组_设定值"() -> (w361:dbl[][])
              n397 = Index Array(array=w360, index=w359) -> (element=w358:bool)
              n398 = case shown="真" w358 {
                tunnel: w359 -> [_ w363]
                tunnel: w361 -> [_ w365]
                tunnel: w357 -> [_ w362]
                frame False {
                }
                frame True {
                  n399 = disable-structure shown="禁用" {
                    frame Disabled {
                      n400 = call "can开关切换.vi"() -> ()  [unwired: 10 in, 1 out]
                    }
                    frame Enabled {
                    }
                  }
                  n401 = case shown="真" TRUE {
                    tunnel: w363 -> [_ w367]
                    tunnel: w365 -> [_ w368]
                    tunnel: w362 -> [_ w366]
                    frame False {
                    }
                    frame True {
                      n402 = local write "第几组数据"(w367) -> ()
                      n403 = for {
                        N: 5 -> [_]
                        tunnel: w367 -> [w373]
                        tunnel: w368 -> [w372]
                        tunnel: w366 -> [w370]
                        i -> [w371]
                        n404 = while {
                          tunnel: w373 -> [w381]
                          tunnel: w372 -> [w380]
                          tunnel: w371 -> [w379]
                          tunnel: w370 -> [w374]
                          stop <- w378 stop-if-true
                          n405 = local read "bSend"() -> (w376:bool)
                          n406 = Wait Until Next ms Multiple(millisecond multiple=u32 10 ("毫秒倍数")) -> ()  [unwired: 1 out]
                          n407 = Not(x=w376) -> (.not. x?=w375:bool)
                          n408 = case shown="真" w375 {
                            tunnel: w381 -> [_ w392]
                            tunnel: w380 -> [_ w391]
                            tunnel: w379 -> [_ w390]
                            tunnel: [w382 FALSE] -> w378
                            tunnel: w374 -> [_ w388]
                            frame False {
                              n409 = local read "bRece"() -> (w383:bool)
                              n410 = case shown="假" w383 {
                                tunnel: [FALSE w385] -> w382
                                frame False {
                                }
                                frame True {
                                n411 = stacked-sequence {
                                tunnel: [_ TRUE] -> w385
                                frame #0 {
                                w386 = FALSE
                                n412 = local write "bSend"(w386) -> ()
                                n413 = local write "bRece"(w386) -> ()
                                }
                                frame #1 {
                                }
                                }
                                }
                              }
                            }
                            frame True {
                              n414 = stacked-sequence {
                                tunnel: w392 -> [w400 _ _]
                                tunnel: w391 -> [w397 _ _]
                                tunnel: w390 -> [w395 _ _]
                                tunnel: w388 -> [_ w408 _]
                                frame #0 {
                                # "PCI板卡下发模拟量数据"
                                n415 = global read "试验配置信息.vi" "设定输出通道"() -> (w399:i32[])
                                n416 = To Long Integer(number=w400) -> (32bit integer=w396:i32)
                                n417 = local write "第几个数据"(w395) -> ()
                                n418 = Index Array(array=w397, index (row)=w396, index (col)=w395) -> (element=w393:dbl)
                                n419 = Index Array(array=w399, index=w396) -> (element=w398:i32)
                                n420 = case shown="1" w398 {
                                tunnel: [w404 w407] -> w394
                                tunnel: w393 -> [w402 w405]
                                frame 0, Default {
                                n421 = Build Array(w402, 0.0) -> (w404:dbl[])
                                }
                                frame 1 {
                                n422 = Build Array(0.0, w405) -> (w407:dbl[])
                                }
                                }
                                n423 = call "Convert to Dynamic Data"("Array"=w394) -> ("Dynamic Data Type"=w401:dynamicdata)  [unwired: 3 out]
                                n424 = call "DAQNavi Assistant"("data in(DDT)"=w401) -> ()  [unwired: 2 in, 17 out]
                                }
                                frame #1 {
                                n425 = local write "同步_1"(1 ("y")) -> ()
                                n426 = Send Notification(notification="NumCheck" ("通知"), notifier=w408) -> ()  [unwired: 1 in, 2 out]
                                }
                                frame #2 {
                                n427 = local write "bSend"(TRUE) -> ()
                                }
                              }
                            }
                          }
                        }
                      }
                    }
                  }
                }
              }
            }
          }
          frame #1 {
            n428 = property on="btn_取消" class="Bool"("DisabledEnum"=T1."Enabled" ("禁用")) -> ()  [unwired: 2 in, 2 out]
          }
        }
      }
    }
    n429 = local read "退出？"() -> (w352:bool)
  }
  n430 = Release Notifier(notifier=w9) -> ()  [unwired: 2 in, 3 out]
  n431 = Obtain Notifier(name (unnamed)=w2, notification data type=w2) -> (notifier out=w1:refnum<notifier>)  [unwired: 2 in, 2 out]
  n432 = while {
    tunnel: w1 -> [w416]
    tunnel: [w415] -> w5
    stop <- w419 stop-if-true
    n433 = Wait Until Next ms Multiple(millisecond multiple=u32 100 ("毫秒倍数")) -> ()  [unwired: 1 out]
    n434 = Wait on Notification(notifier=w416, timeout in ms (-1)=10 ("超时毫秒(-1)")) -> (notifier out=w415:refnum<notifier>, notification=w414:string)  [unwired: 2 in, 2 out]
    n435 = Equal?(x=w414, y="NumCheck" ("通知")) -> (x = y?=w417:bool)
    n436 = case shown="真" w417 {
      frame False {
      }
      frame True {
        n437 = call "DAQNavi Assistant2"() -> ("error out"=w424:errorcluster, "data out(DDT)"=w425:dynamicdata)  [unwired: 2 in, 16 out]
        n438 = Unbundle By Name(w424) -> ("status"=w422:bool)
        n439 = case shown="真" w422 {
          frame False {
          }
          frame True {
            n440 = call "超时"() -> ()  [unwired: 10 in, 2 out]
            n441 = local write "同步_1"(0 ("同步_1")) -> ()
          }
        }
        n442 = call "从动态数据转换"("Dynamic Data Type"=w425) -> ("Array"=w426:dbl[])  [unwired: 3 in]
        n443 = To Single Precision Float(number=w426) -> (single precision float=w421:sgl[])
        n444 = Not(x=w422) -> (.not. x?=w423:bool)
        n445 = case shown="真" w423 {
          tunnel: w421 -> [_ w428]
          frame False {
          }
          frame True {
            n446 = stacked-sequence {
              tunnel: w428 -> [w454 _ _ _ _]
              frame #0 {
                n447 = global read "试验配置信息.vi" "设定输入通道"() -> (w453:i32[])
                n448 = local read "第几组数据"() -> (w452:i32)
                n449 = local read "第几组数据"() -> (w439:i32)
                n450 = global read "试验配置信息.vi" "允许误差"() -> (w440:dbl[])
                n451 = global read "试验配置信息.vi" "参数A1"() -> (w448:dbl[])
                n452 = global read "试验配置信息.vi" "参数A2"() -> (w447:dbl[])
                n453 = global read "试验配置信息.vi" "Max"() -> (w441:dbl[])
                n454 = global read "试验配置信息.vi" "min"() -> (w442:dbl[])
                n455 = local read "第几个数据"() -> (w450:i32)
                n456 = local read "数组_设定值"() -> (w464:dbl[][])
                n457 = Index Array(array=w453, index=w452) -> (element=w451:i32)
                n458 = Index Array(array=w454, index=w451) -> (element=w430:sgl)
                n459 = Index Array(array=w441, index=w439) -> (element=w438:dbl)
                n460 = Index Array(array=w442, index=w439) -> (element=w437:dbl)
                n461 = Index Array(array=w448, index=w439) -> (element=w446:dbl)
                n462 = Index Array(array=w447, index=w439) -> (element=w445:dbl)
                n463 = Index Array(array=w440, index=w439) -> (element=w434:dbl)
                n464 = Subtract(x=w438, y=w437) -> (x-y=w436:dbl)
                n465 = local read "Analog_back"() -> (w458:string[][])
                n466 = local read "第几个数据"() -> (w455:i32)
                n467 = Absolute Value(x=w436) -> (abs(x)=w435:dbl)
                n468 = Index Array(array=w464, index (row)=w439, index (col)=w450) -> (element=w449:dbl)
                n469 = local read "数组_选择"() -> (w444:bool[])
                n470 = Number To Fractional String(number=w430, precision (6)=i16 3 ("精度(6)")) -> (F-format string=w429:string)  [unwired: 2 in]
                n471 = call "函数公式.vi"("参数 b"=w445, "参数 a"=w446, "设定值 1"=w449) -> ("y"=w443:dbl)  [unwired: 5 in, 1 out]
                n472 = Replace Array Subset(array=w458, new element=w429, index (row)=w452, index (col)=w455) -> (w457:string[][])
                n473 = call "误差计算.vi"("选择?"=w444, "允许误差"=w434, "模拟量量程范围"=w435, "设定值_1"=w443, "反馈值_1"=w430) -> ("字符串_误差_1"=w432:string, "合格_1?"=w433:bool)  [unwired: 4 in, 1 out]
                n474 = local write "Analog_back"(w457) -> ()
                n475 = local read "第几个数据"() -> (w456:i32)
                n476 = local read "Analog_WC"() -> (w463:string[][])
                n477 = local read "第几组数据"() -> (w461:i32)
                n478 = Replace Array Subset(array=w463, new element=w432, index (row)=w461, index (col)=w456) -> (w462:string[][])
                n479 = local read "合格？"() -> (w459:bool[][])
                n480 = local write "Analog_WC"(w462) -> ()
                n481 = Replace Array Subset(array=w459, new element=w433, index (row)=w461, index (col)=w456) -> (w460:bool[][])
                n482 = local write "合格？"(w460) -> ()
              }
              frame #1 {
                n483 = local read "合格？"() -> (w469:bool[][])
                n484 = local read "第几组数据"() -> (w466:i32)
                n485 = Index Array(array=w469, index (row)=w466) -> (element=w471:bool[])  [unwired: 1 in]
                n486 = And Array Elements(Boolean array=w471) -> (logical AND=w468:bool)
                n487 = local read "数组_选择"() -> (w467:bool[])
                n488 = Index Array(array=w467, index=w466) -> (element=w465:bool)
                n489 = case shown="真" w465 {
                  tunnel: [cluster{u32, u32}[] [{12369084, 12369084}] w474] -> w470
                  tunnel: w468 -> [_ w473]
                  frame False {
                  }
                  frame True {
                    n490 = case shown="真" w473 {
                      tunnel: [cluster{u32, u32}[] [{16730410, 16711680}] cluster{u32, u32}[] [{61205, 6618880}]] -> w474
                      frame False {
                      }
                      frame True {
                      }
                    }
                  }
                }
                n491 = case shown="31" w466 {
                  tunnel: w470 -> [w477 w478 w479 w480 w481 w482 w483 w484 w485 w486 w487 w488 w489 w490 w491 w492 w493 w494 w495 w496 w497 w498 w499 w500 w501 w502 w503 w504 w505 w506 w507 w508]
                  frame 0, Default {
                    n492 = property on="light_1" class="Bool (严格)"("Colors [4]"=w477) -> ()  [unwired: 2 in, 2 out]
                  }
                  frame 1 {
                    n493 = property on="light_2" class="Bool (严格)"("Colors [4]"=w478) -> ()  [unwired: 2 in, 2 out]
                  }
                  frame 2 {
                    n494 = property on="light_3" class="Bool (严格)"("Colors [4]"=w479) -> ()  [unwired: 2 in, 2 out]
                  }
                  frame 3 {
                    n495 = property on="light_4" class="Bool (严格)"("Colors [4]"=w480) -> ()  [unwired: 2 in, 2 out]
                  }
                  frame 4 {
                    n496 = property on="light_5" class="Bool (严格)"("Colors [4]"=w481) -> ()  [unwired: 2 in, 2 out]
                  }
                  frame 5 {
                    n497 = property on="light_6" class="Bool (严格)"("Colors [4]"=w482) -> ()  [unwired: 2 in, 2 out]
                  }
                  frame 6 {
                    n498 = property on="light_7" class="Bool (严格)"("Colors [4]"=w483) -> ()  [unwired: 2 in, 2 out]
                  }
                  frame 7 {
                    n499 = property on="light_8" class="Bool (严格)"("Colors [4]"=w484) -> ()  [unwired: 2 in, 2 out]
                  }
                  frame 8 {
                    n500 = property on="light_9" class="Bool (严格)"("Colors [4]"=w485) -> ()  [unwired: 2 in, 2 out]
                  }
                  frame 9 {
                    n501 = property on="light_10" class="Bool (严格)"("Colors [4]"=w486) -> ()  [unwired: 2 in, 2 out]
                  }
                  frame 10 {
                    n502 = property on="light_11" class="Bool (严格)"("Colors [4]"=w487) -> ()  [unwired: 2 in, 2 out]
                  }
                  frame 11 {
                    n503 = property on="light_12" class="Bool (严格)"("Colors [4]"=w488) -> ()  [unwired: 2 in, 2 out]
                  }
                  frame 12 {
                    n504 = property on="light_13" class="Bool (严格)"("Colors [4]"=w489) -> ()  [unwired: 2 in, 2 out]
                  }
                  frame 13 {
                    n505 = property on="light_14" class="Bool (严格)"("Colors [4]"=w490) -> ()  [unwired: 2 in, 2 out]
                  }
                  frame 14 {
                    n506 = property on="light_15" class="Bool (严格)"("Colors [4]"=w491) -> ()  [unwired: 2 in, 2 out]
                  }
                  frame 15 {
                    n507 = property on="light_16" class="Bool (严格)"("Colors [4]"=w492) -> ()  [unwired: 2 in, 2 out]
                  }
                  frame 16 {
                    n508 = property on="light_17" class="Bool (严格)"("Colors [4]"=w493) -> ()  [unwired: 2 in, 2 out]
                  }
                  frame 17 {
                    n509 = property on="light_18" class="Bool (严格)"("Colors [4]"=w494) -> ()  [unwired: 2 in, 2 out]
                  }
                  frame 18 {
                    n510 = property on="light_19" class="Bool (严格)"("Colors [4]"=w495) -> ()  [unwired: 2 in, 2 out]
                  }
                  frame 19 {
                    n511 = property on="light_20" class="Bool (严格)"("Colors [4]"=w496) -> ()  [unwired: 2 in, 2 out]
                  }
                  frame 20 {
                    n512 = property on="light_21" class="Bool (严格)"("Colors [4]"=w497) -> ()  [unwired: 2 in, 2 out]
                  }
                  frame 21 {
                    n513 = property on="light_22" class="Bool (严格)"("Colors [4]"=w498) -> ()  [unwired: 2 in, 2 out]
                  }
                  frame 22 {
                    n514 = property on="light_23" class="Bool (严格)"("Colors [4]"=w499) -> ()  [unwired: 2 in, 2 out]
                  }
                  frame 23 {
                    n515 = property on="light_24" class="Bool (严格)"("Colors [4]"=w500) -> ()  [unwired: 2 in, 2 out]
                  }
                  frame 24 {
                    n516 = property on="light_25" class="Bool (严格)"("Colors [4]"=w501) -> ()  [unwired: 2 in, 2 out]
                  }
                  frame 25 {
                    n517 = property on="light_26" class="Bool (严格)"("Colors [4]"=w502) -> ()  [unwired: 2 in, 2 out]
                  }
                  frame 26 {
                    n518 = property on="light_27" class="Bool (严格)"("Colors [4]"=w503) -> ()  [unwired: 2 in, 2 out]
                  }
                  frame 27 {
                    n519 = property on="light_28" class="Bool (严格)"("Colors [4]"=w504) -> ()  [unwired: 2 in, 2 out]
                  }
                  frame 28 {
                    n520 = property on="light_29" class="Bool (严格)"("Colors [4]"=w505) -> ()  [unwired: 2 in, 2 out]
                  }
                  frame 29 {
                    n521 = property on="light_30" class="Bool (严格)"("Colors [4]"=w506) -> ()  [unwired: 2 in, 2 out]
                  }
                  frame 30 {
                    n522 = property on="light_31" class="Bool (严格)"("Colors [4]"=w507) -> ()  [unwired: 2 in, 2 out]
                  }
                  frame 31 {
                    n523 = property on="light_32" class="Bool (严格)"("Colors [4]"=w508) -> ()  [unwired: 2 in, 2 out]
                  }
                }
              }
              frame #2 {
                n524 = local read "第几组数据"() -> (w510:i32)
                n525 = local read "第几个数据"() -> (w513:i32)
                n526 = local read "合格？"() -> (w514:bool[][])
                n527 = local read "数组_选择"() -> (w512:bool[])
                n528 = Index Array(array=w514, index (row) #1=w510, index (col) #1=w513, index (col) #2=w513) -> (element #1=w511:bool)  [unwired: 1 in, 1 out]
                n529 = Index Array(array=w512, index=w510) -> (element=w509:bool)
                n530 = case shown="真" w509 {
                  tunnel: w513 -> [_ w518]
                  tunnel: w511 -> [_ w517]
                  tunnel: w510 -> [_ w516]
                  frame False {
                  }
                  frame True {
                    n531 = call "误差表格颜色.vi"("合格？"=w517, "第几组"=w516) -> ("颜色"=w515:u32)  [unwired: 9 in]
                    n532 = Bundle("第几组数据"=w516, "第几个数据"=w518) -> (w520:cluster{"第几组数据":i32, "第几个数据":i32})  [unwired: 1 in]
                    n533 = property on="Analog_WC" class="Tbl (严格)"("Active Cell"=w520) -> (error out=w519:errorcluster)  [unwired: 2 in, 1 out]
                    n534 = property on="Analog_WC" class="Tbl (严格)"(error in=w519, "Cell BG Color"=w515) -> ()  [unwired: 1 in, 2 out]
                  }
                }
              }
              frame #3 {
                n535 = Wait Until Next ms Multiple(millisecond multiple=u32 100 ("毫秒倍数")) -> ()  [unwired: 1 out]
              }
              frame #4 {
                n536 = local write "bRece"(TRUE) -> ()
              }
            }
          }
        }
      }
    }
    n537 = local read "退出？"() -> (w419:bool)
  }
  n538 = Release Notifier(notifier=w5) -> ()  [unwired: 2 in, 3 out]
